vi "Line Stream To File.vi"(8 "file path":path, 11 "lines in":T1) -> ()   [LabVIEW 2023]
uses:
  <extravilib>/ChannelInstances/Stream-str/)Channel.ctl
  <extravilib>/ChannelInstances/Stream-str/Read With Abort.vi
  <extravilib>/ChannelInstances/Stream-str/EndpointRead.vi
  <extravilib>/ChannelInstances/Stream-str/)Channel.vi
  <resource>/ChannelSupport/_ChannelSupport/WaitIfNeeded.vi
  <extravilib>/ChannelInstances/Stream-str.lvlib
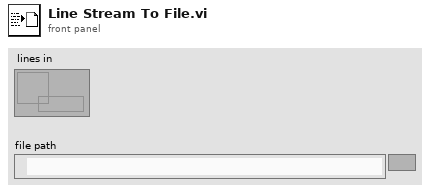
[diagram p1: front panel]
types:
  T1 = typedef "Stream-str.lvlib/)Channel.ctl" = refnum<queue>
  T2 = enum16{"open", "replace", "create", "open or create", "replace or create", "replace or create with confirmation"}
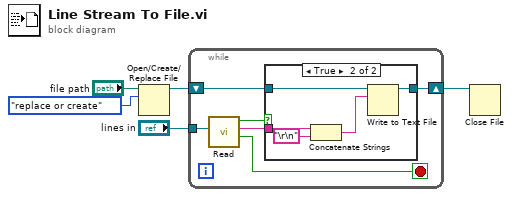
[diagram p0: block diagram]
diagram:
  n1 = Open/Create/Replace File(file path (use dialog)="file path", operation (0:open)=T2."replace or create") -> (refnum out=w3:refnum<file>)  [unwired: 4 in, 2 out]
  n2 = while {
    shift-right: [w10] -> w1
    shift-left: w3 -> [w11]
    tunnel: "lines in" -> [w9]
    stop <- w6 stop-if-true
    n3 = call <extravilib>:"Read.vi"("channel"=w9) -> ("last element?"=w6:bool, "element"=w8:string, "element valid?"=w7:bool)  [unwired: 6 in, 2 out]
    n4 = case shown="True" w7 {
      tunnel: w11 -> [w12 w17]
      tunnel: [w12 w16] -> w10
      tunnel: w8 -> [_ w15]
      frame False {
      }
      frame True {
        n5 = Concatenate Strings(w15, "\r\n") -> (w14:string)
        n6 = Write to Text File(file (use dialog)=w17, text=w14) -> (refnum out=w16:refnum<file>)  [unwired: 2 in, 2 out]
      }
    }
  }
  n7 = Close File(refnum=w1) -> ()  [unwired: 1 in, 2 out]
